vi "ukol3.vi"() -> ()   [LabVIEW 2022 SP3]
panel:
  out "Array 2":string[](array[string])
  out "32bit integer":i32[](array[numeric])
  out "size(s)":i32
  in  "Array":dbl[](array[numeric])
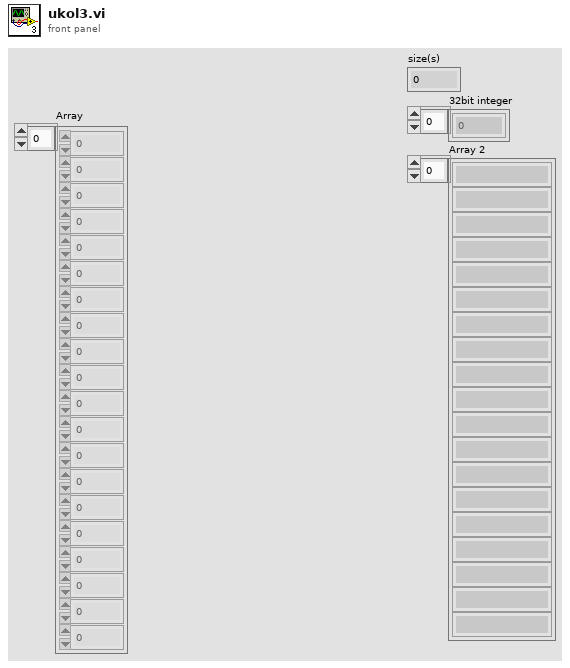
[diagram p1: front panel]
types:
  T1 = enum16{"open", "replace", "create", "open or create", "replace or create", "replace or create with confirmation"}
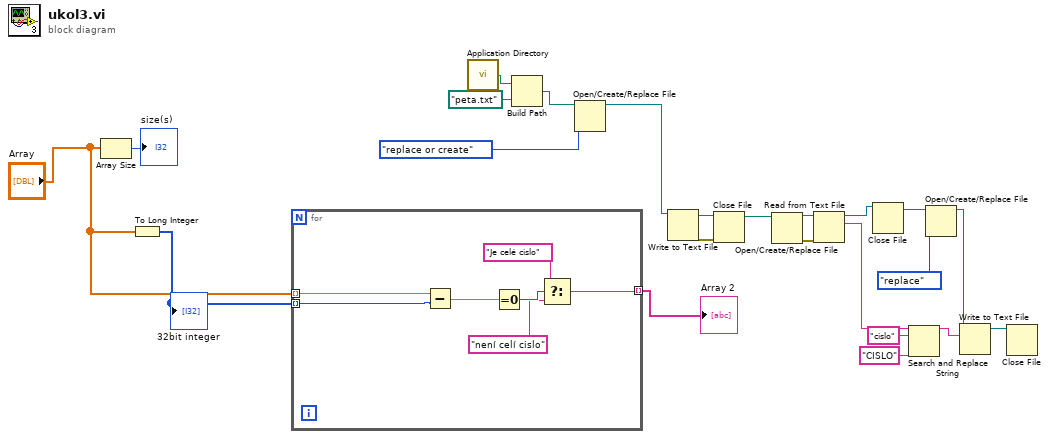
[diagram p0: block diagram]
diagram:
  n1 = Array Size(array="Array") -> (size(s)=→"size(s)":i32)
  n2 = To Long Integer(number="Array") -> (32bit integer=w21:i32[])
  "32bit integer" <- w21
  n3 = for {
    tunnel: "Array" -> [w30] mode=indexing
    tunnel: w21 -> [w29] mode=indexing
    tunnel: [w24] -> w1 mode=indexing
    n4 = Subtract(x=w30, y=w29) -> (x-y=w28:dbl)
    n5 = Equal To 0?(x=w28) -> (x = 0?=w27:bool)
    n6 = Select(t="Je celé cislo", s=w27, f="není celí cislo") -> (s? t:f=w24:string)
  }
  "Array 2" <- w1
  n7 = call <vilib>:"Application Directory.vi"() -> ("Application Directory"=w3:path)
  n8 = Build Path(base path=w3, name or relative path=path "peta.txt") -> (appended path=w2:path)
  n9 = Open/Create/Replace File(file path (use dialog)=w2, operation (0:open)=T1."replace or create") -> (refnum out=w6:refnum<file>)  [unwired: 4 in, 2 out]
  n10 = Write to Text File(file (use dialog)=w6) -> (refnum out=w20:refnum<file>, error out=w19:errorcluster)  [unwired: 3 in, 1 out]
  n11 = Close File(refnum=w20, error in=w19) -> (path=w18:path)  [unwired: 1 out]
  n12 = Open/Create/Replace File(file path (use dialog)=w18) -> (refnum out=w16:refnum<file>, error out=w17:errorcluster)  [unwired: 5 in, 1 out]
  n13 = Read from Text File(file (use dialog)=w16, error in=w17) -> (refnum out=w11:refnum<file>, text=w15:string)  [unwired: 2 in, 2 out]
  n14 = Close File(refnum=w11) -> (path=w10:path)  [unwired: 1 in, 1 out]
  n15 = Search and Replace String(input string=w15, search string="cislo", replace string="CISLO" ("replace string (\"\")")) -> (result string=w12:string)  [unwired: 5 in, 3 out]
  n16 = Open/Create/Replace File(file path (use dialog)=w10, operation (0:open)=T1."replace") -> (refnum out=w8:refnum<file>)  [unwired: 4 in, 2 out]
  n17 = Write to Text File(file (use dialog)=w8, text=w12) -> (refnum out=w7:refnum<file>)  [unwired: 2 in, 2 out]
  n18 = Close File(refnum=w7) -> ()  [unwired: 1 in, 2 out]
